vi "ToteStoppercontrol.vi"(0 "Right moving":bool, 1 "Left moving?":bool, 2 "Last True":i32, 5 "outputY":dbl, 7 "ToteRightPull":bool, 9 "outputX":dbl, 12 "ToteLeftspit":bool, 13 "ToteRigthspit":bool, 14 "ToteLeftPull":bool) -> ()   [LabVIEW 2014]
uses:
  <vilib>/Rock Robotics/WPI/Relay/WPI_RelayValue.ctl
  Robot Values.vi
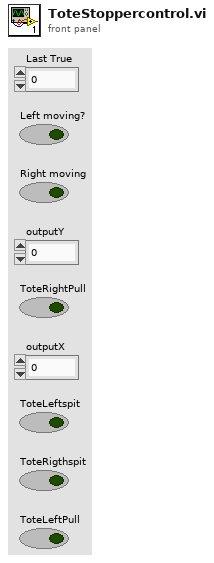
[diagram p1: front panel]
types:
  T1 = typedef "WPI_RelayValue.ctl" = enum16{"Off", "On", "Forward", "Reverse"}
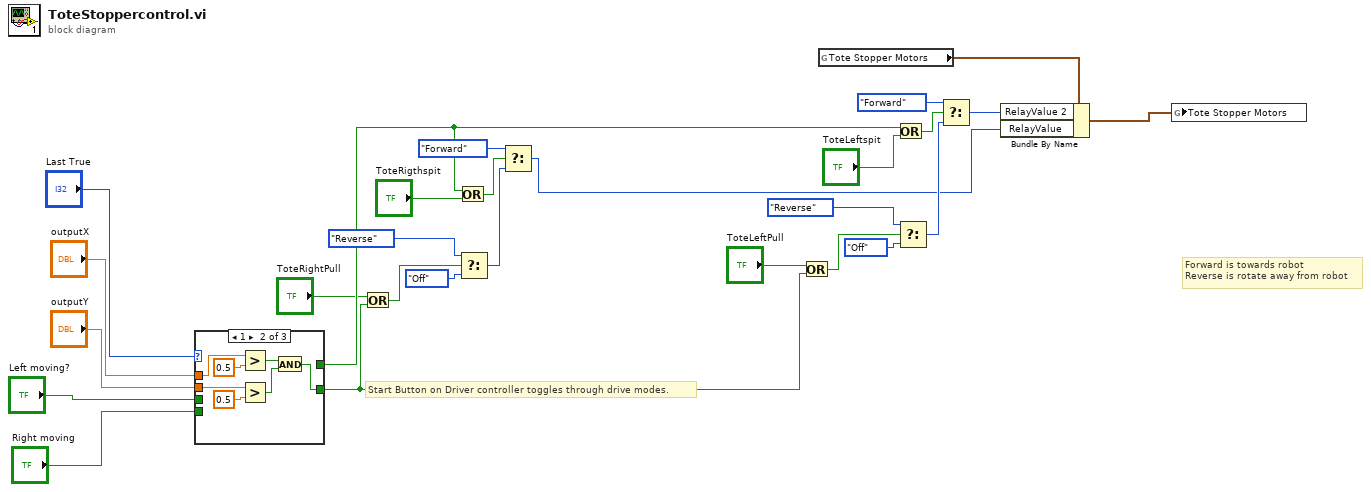
[diagram p0: block diagram]
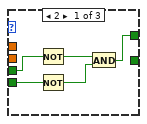
[diagram p2: hidden frame]
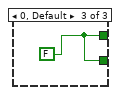
[diagram p3: hidden frame]
diagram:
  # "Forward is towards robot\nReverse is rotate away from robot"
  # "Start Button on Driver controller toggles through drive modes."
  n1 = case shown="1" "Last True" {
    tunnel: "Left moving?" -> [w32 _ _]
    tunnel: "Right moving" -> [w31 _ _]
    tunnel: [_ w33 w40] -> w22
    tunnel: "outputY" -> [_ w38 _]
    tunnel: "outputX" -> [_ w39 _]
    tunnel: [w28 _ w40] -> w27
    frame 2 {
      n2 = Not(x=w32) -> (.not. x?=w29:bool)
      n3 = Not(x=w31) -> (.not. x?=w30:bool)
      n4 = And(x=w29, y=w30) -> (x .and. y?=w28:bool)
    }
    frame 1 {
      n5 = Greater?(x=w39, y=0.5) -> (0:w35:bool)
      n6 = Greater?(x=w38, y=0.5) -> (0:w34:bool)
      n7 = And(x=w35, y=w34) -> (x .and. y?=w33:bool)
    }
    frame 0, Default {
      w40 = FALSE
    }
  }
  n8 = Or(x="ToteRightPull", y=w22) -> (x .or. y?=w20:bool)
  n9 = Or(x=w27, y="ToteRigthspit") -> (x .or. y?=w25:bool)
  n10 = Select(t=WPI_RelayValue."Reverse" ("RelayValue"), s=w20, f=WPI_RelayValue."Off" ("RelayValue")) -> (s? t:f=w12:T1)
  n11 = Select(t=WPI_RelayValue."Forward" ("RelayValue"), s=w25, f=w12) -> (s? t:f=w1:T1)
  n12 = Or(x="ToteLeftPull", y=w22) -> (x .or. y?=w21:bool)
  n13 = global read "Robot Values.vi" "Tote Stopper Motors"() -> (w2:cluster{"RelayValue":T1, "RelayValue 2":T1})
  n14 = Or(x=w27, y="ToteLeftspit") -> (x .or. y?=w26:bool)
  n15 = Select(t=WPI_RelayValue."Reverse" ("RelayValue"), s=w21, f=WPI_RelayValue."Off" ("RelayValue")) -> (s? t:f=w9:T1)
  n16 = Select(t=WPI_RelayValue."Forward" ("RelayValue"), s=w26, f=w9) -> (s? t:f=w8:T1)
  n17 = Bundle By Name(cluster=w2, "RelayValue 2"=w8, "RelayValue"=w1) -> (w3:cluster{"RelayValue":T1, "RelayValue 2":T1})
  n18 = global write "Robot Values.vi" "Tote Stopper Motors"(w3) -> ()
